vi "raster_scan_ground_shutter.vi"() -> ()   [LabVIEW 2013] (continued)
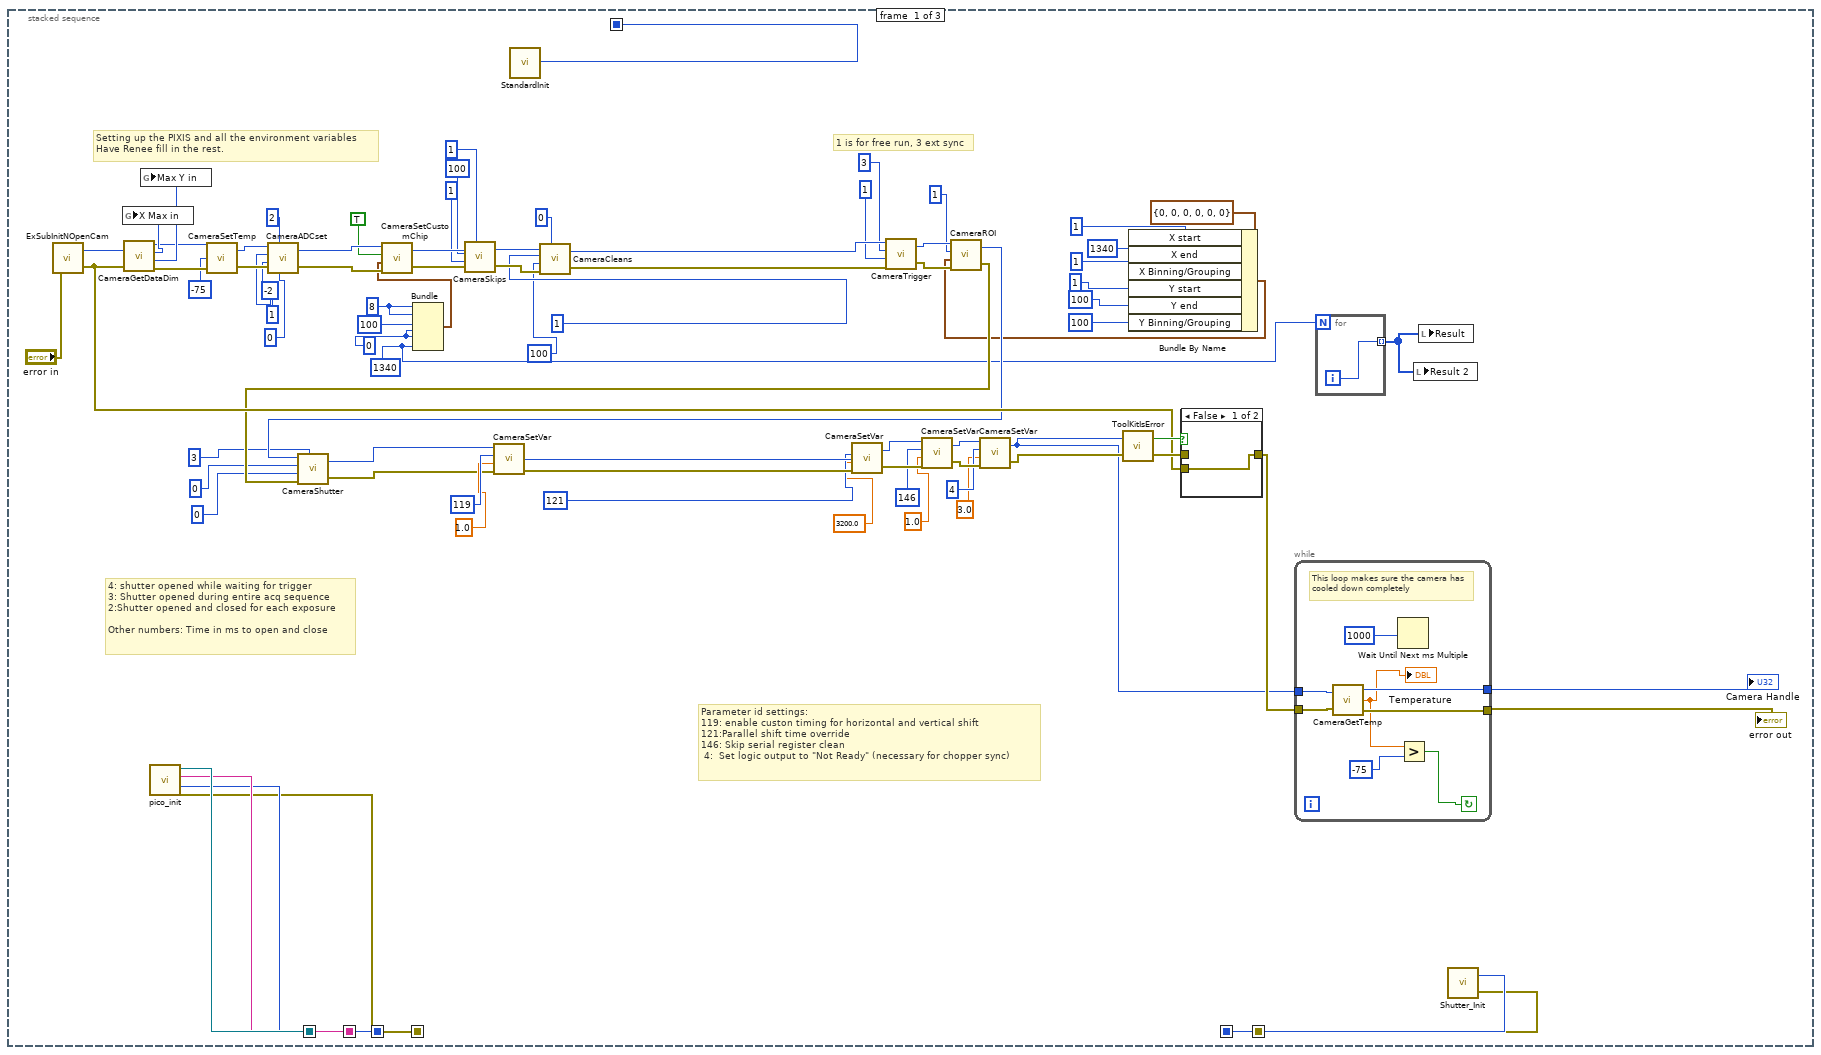
[diagram p2: hidden frame]
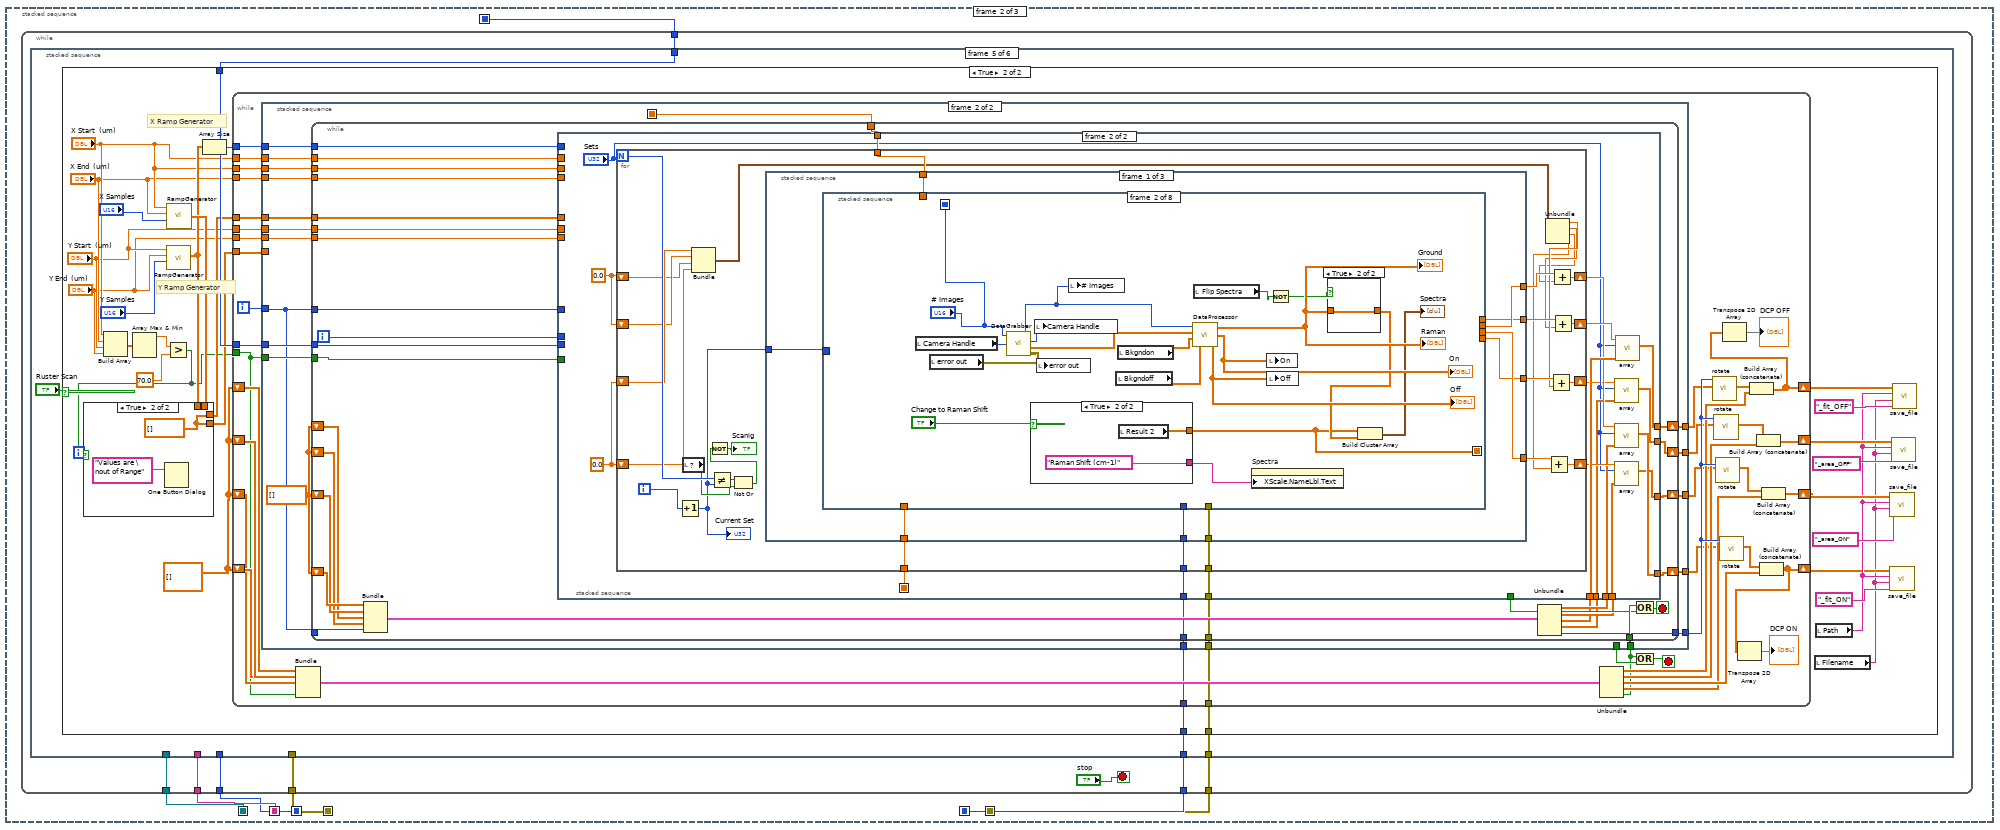
[diagram p4: hidden frame]
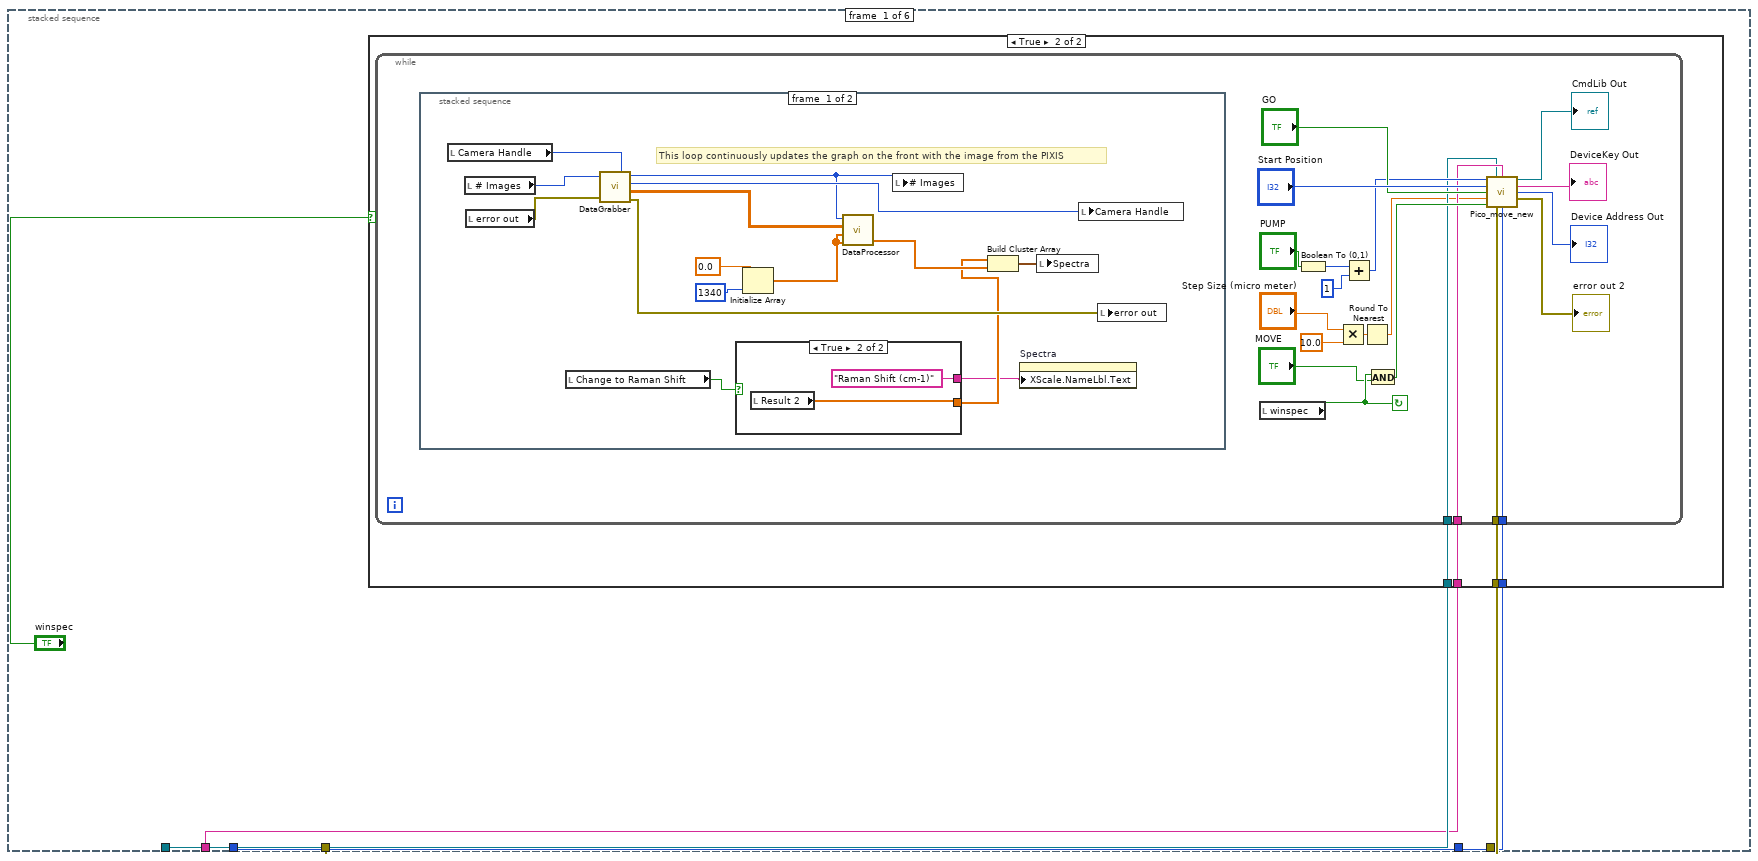
[diagram p5: hidden frame]
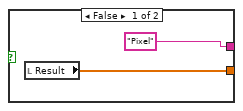
[diagram p7: hidden frame]
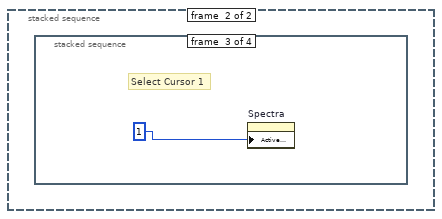
[diagram p8: hidden frame]
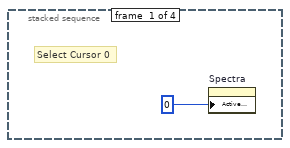
[diagram p9: hidden frame]
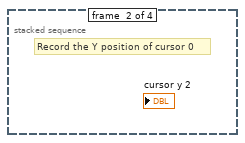
[diagram p10: hidden frame]
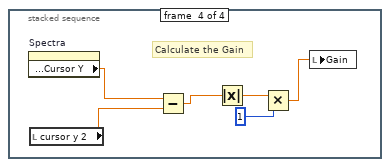
[diagram p11: hidden frame]
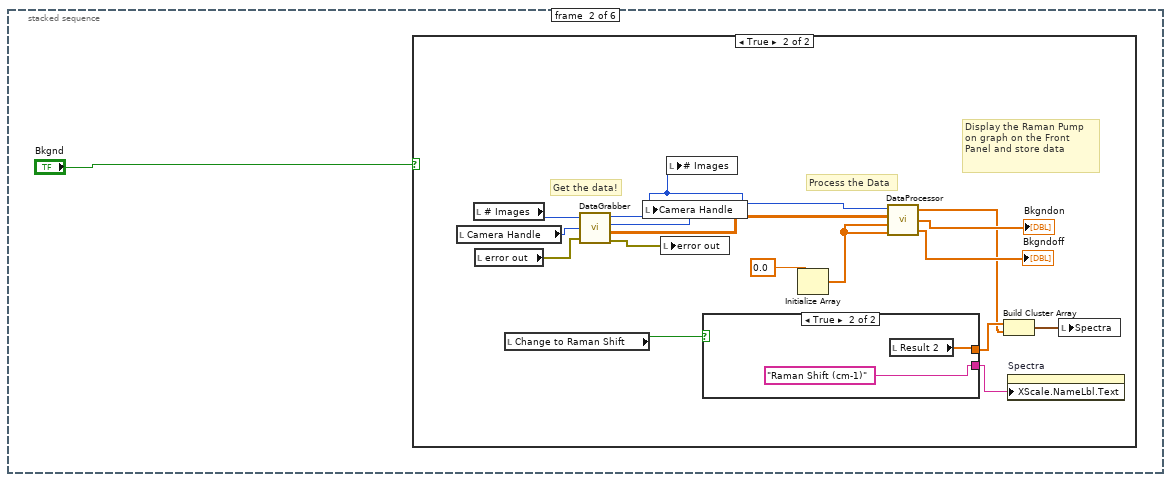
[diagram p12: hidden frame]
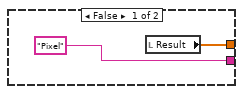
[diagram p14: hidden frame]
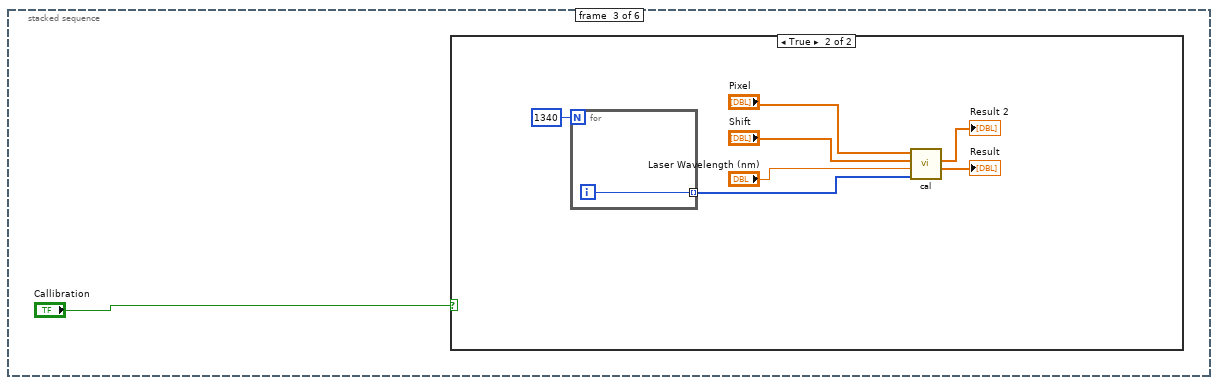
[diagram p15: hidden frame]
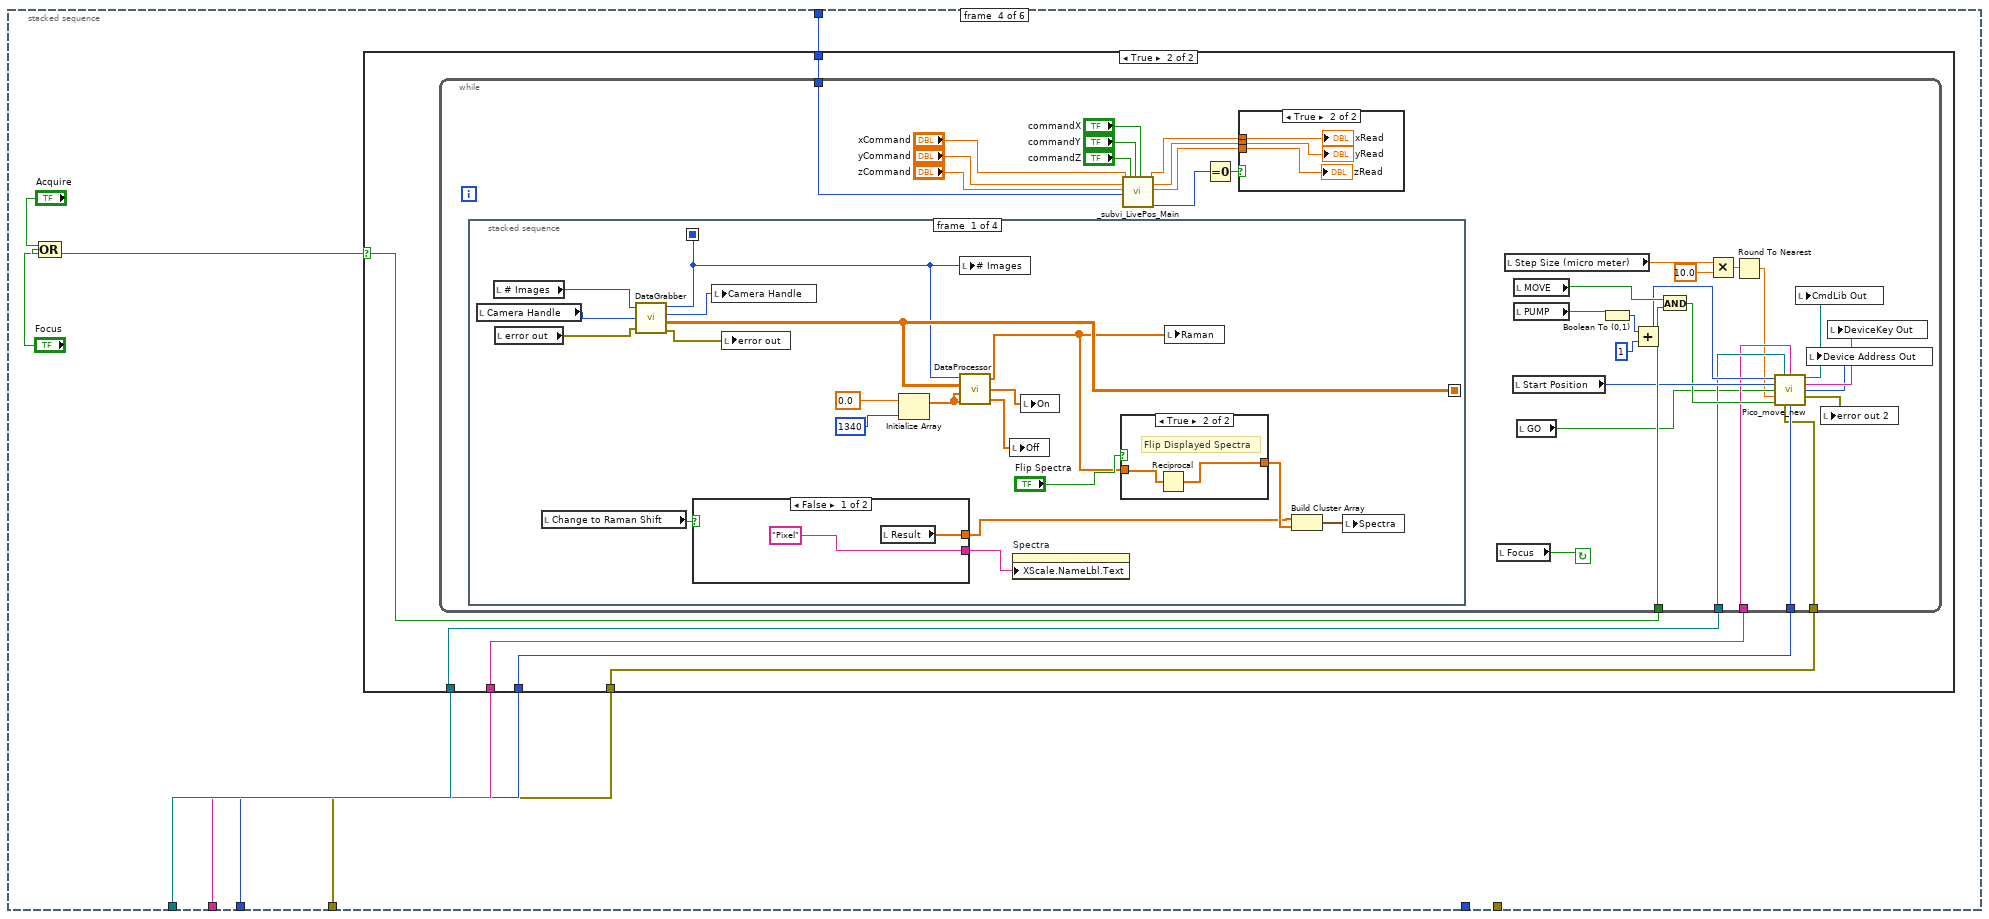
[diagram p17: hidden frame]
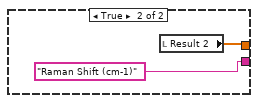
[diagram p20: hidden frame]
                  n154 = call "Pico_move_new.vi"("Motor"=w239, "CmdLib Out"=w236, "DeviceKey Out"=w235, "Start Position"=w238, "Boolean 2"=w232, "Relative Steps"=w224, "Boolean"=w237, "error out"=w233, "Device Address Out"=w234) -> ("CmdLib Out"=w231:refnum<k24>, "DeviceKey Out"=w230:string, "Device Address Out"=w229:i32, "error out 2"=w228:errorcluster)  [unwired: 3 in]
                  n155 = local write "CmdLib Out"(w231) -> ()
                  n156 = local write "Device Address Out"(w229) -> ()
                  n157 = local write "error out 2"(w228) -> ()
                  n158 = local write "DeviceKey Out"(w230) -> ()
                }
              }
            }
          }
          frame #4 {
            n159 = case shown="True" "Ruster Scan" {
              tunnel: w326 -> [_ w356]
              tunnel: w325 -> [_ w330]
              tunnel: w324 -> [_ w329]
              frame False {
              }
              frame True {
                w348 = dbl[][] []
                # "X Ramp Generator"
                # "Y Ramp Generator"
                n160 = Build Array("X Start  (um)", "X End  (um)", "Y Start  (um)", "Y End  (um)") -> (w347:dbl[])
                n161 = Array Max & Min(array=w347) -> (max value=w341:dbl)  [unwired: 3 out]
                n162 = call "RampGenerator.vi"("Number of Positions"="Y Samples", "End  (um)"="Y End  (um)", "Start  (um)"="Y Start  (um)") -> ("Array"=w350:dbl[])  [unwired: 1 in]
                n163 = Greater?(x=w341, y=70.0) -> (0:w331:bool)
                n164 = call "RampGenerator.vi"("Number of Positions"="X Samples", "End  (um)"="X End  (um)", "Start  (um)"="X Start  (um)") -> ("Array"=w351:dbl[])  [unwired: 1 in]
                n165 = case shown="True" w331 {
                  tunnel: [w358 w360] -> w352
                  tunnel: w350 -> [w358 _]
                  tunnel: [w357 w360] -> w353
                  tunnel: w351 -> [w357 _]
                  frame False {
                  }
                  frame True {
                    w360 = dbl[] [] ("Array")
                    n166 = One Button Dialog(message="Values are \nout of Range") -> ()  [unwired: 1 in, 1 out]
                  }
                }
                n167 = Array Size(array=w350) -> (size(s)=w349:i32)
                n168 = while {
                  tunnel: w352 -> [w400]
                  tunnel: w356 -> [w399]
                  tunnel: w353 -> [w398]
                  tunnel: "X Start  (um)" -> [w397]
                  shift-right: [w392] -> w332
                  shift-left: w348 -> [w375]
                  shift-right: [w394] -> w336
                  shift-left: w348 -> [w374]
                  tunnel: w331 -> [w365]
                  tunnel: w349 -> [w389]
                  tunnel: "X Start  (um)" -> [w388]
                  tunnel: "X End  (um)" -> [w387]
                  tunnel: "Y Start  (um)" -> [w386]
                  tunnel: "Y End  (um)" -> [w385]
                  shift-right: [w380] -> w337
                  shift-left: w348 -> [w376]
                  shift-right: [w378] -> w340
                  shift-left: w348 -> [w377]
                  tunnel: w330 -> [w362]
                  tunnel: w329 -> [w361]
                  i -> [w396]
                  stop <- w363 stop-if-true
                  n169 = Bundle(w377, w376, w375, w374, w365) -> (w373:T3)  [unwired: 1 in]
                  n170 = Unbundle(w373) -> (w372:dbl[][], w369:dbl[][], w371:dbl[][], w370:dbl[][], w364:bool)
                  n171 = stacked-sequence {
                    seq-local: [w402 _] -> [_ w428]
                    tunnel: w400 -> [w406 _]
                    tunnel: w396 -> [w404 w415]
                    tunnel: w399 -> [w405 w429]
                    tunnel: w398 -> [_ w431]
                    tunnel: w397 -> [_ w430]
                    tunnel: [w403 _] -> w391
                    tunnel: [_ w427] -> w368
                    tunnel: [_ w426] -> w367
                    tunnel: [_ w414] -> w384
                    tunnel: w365 -> [_ w425]
                    tunnel: w364 -> [_ w424]
                    tunnel: w389 -> [_ w423]
                    tunnel: w388 -> [_ w422]
                    tunnel: w387 -> [_ w421]
                    tunnel: w386 -> [_ w420]
                    tunnel: w385 -> [_ w419]
                    tunnel: [_ w417] -> w366
                    tunnel: [_ w416] -> w383
                    tunnel: w362 -> [_ w413]
                    tunnel: w361 -> [_ w412]
                    frame #0 {
                      w409 = 2  # Y AXIS
                      # "Step the Y axis"
                      n172 = Array Size(array=w406) -> (size(s)=w401:i32)
                      n173 = Index Array(array=w406, index=w404) -> (element=w407:dbl)
                      n174 = Increment(x=w404) -> (x+1=w408:i32)
                      n175 = Subtract(x=w401, y=w408) -> (x-y=w411:i32)
                      n176 = Equal To 0?(x=w411) -> (x = 0?=w403:bool)
                      n177 = call "WriteReadN.vi"("Handle"=w405, "Axis"=w409, "Delay (ms)"="Y Delay (ms)", "Move to (um)"=w407) -> ("Current Position (um)"=w402:dbl)
                      "Y Position (um)" <- w402
                    }
                    frame #1 {
                      w418 = dbl[] []
                      n178 = while {
                        tunnel: w431 -> [w463]
                        tunnel: w430 -> [w462]
                        tunnel: w429 -> [w460]
                        tunnel: w428 -> [w459]
                        tunnel: w415 -> [w446]
                        shift-right: [w458] -> w427
                        shift-left: w418 -> [w445]
                        shift-right: [w457] -> w426
                        shift-left: w418 -> [w444]
                        tunnel: w425 -> [w456]
                        tunnel: w424 -> [w454]
                        tunnel: w423 -> [w453]
                        tunnel: w422 -> [w452]
                        tunnel: w421 -> [w451]
                        tunnel: w420 -> [w450]
                        tunnel: w419 -> [w449]
                        shift-right: [w448] -> w417
                        shift-left: w418 -> [w443]
                        shift-right: [w447] -> w416
                        shift-left: w418 -> [w438]
                        tunnel: w415 -> [w435]
                        tunnel: [w434] -> w414
                        tunnel: w413 -> [w433]
                        tunnel: w412 -> [w432]
                        i -> [w461]
                        stop <- w455 stop-if-true
                        n179 = Bundle(w445, w444, w438, w443, w435) -> (w441:cluster{dbl[], dbl[], dbl[], dbl[], i32})  [unwired: 1 in]
                        n180 = Unbundle(w441) -> (w440:dbl[], w439:dbl[], w437:dbl[], w436:dbl[], w434:i32)
                        n181 = stacked-sequence {
                          seq-local: [w481 _] -> [_ w520]
                          tunnel: w463 -> [w486 _]
                          tunnel: w462 -> [_ _]
                          tunnel: w461 -> [w477 _]
                          tunnel: w460 -> [w494 _]
                          tunnel: [w493 _] -> w442
                          tunnel: w459 -> [w492 w521]
                          tunnel: w446 -> [w479 _]
                          tunnel: w440 -> [_ w512]
                          tunnel: [_ w511] -> w458
                          tunnel: [_ w505] -> w457
                          tunnel: w439 -> [_ w514]
                          tunnel: w456 -> [_ _]
                          tunnel: w453 -> [w480 _]
                          tunnel: w452 -> [w469 _]
                          tunnel: w451 -> [w468 _]
                          tunnel: w450 -> [w466 _]
                          tunnel: w449 -> [w467 _]
                          tunnel: w436 -> [_ w509]
                          tunnel: [_ w508] -> w448
                          tunnel: w437 -> [_ w517]
                          tunnel: [_ w515] -> w447
                          tunnel: w433 -> [_ w504]
                          tunnel: w432 -> [_ w503]
                          frame #0 {
                            w495 = 1  # X AXIS
                            # "Step the X axis"
                            n182 = Quotient & Remainder(x=w479, y=2) -> (x-y*floor(x/y)=w490:i32)  [unwired: 1 out]
                            n183 = Array Size(array=w486) -> (size(s)=w478:i32)
                            n184 = Equal?(x=w490, y=0) -> (x = y?=w483:bool)
                            n185 = Multiply(x=w478, y=w479) -> (x*y=w475:i32)
                            n186 = Increment(x=w477) -> (x+1=w476:i32)
                            n187 = Subtract(x=w478, y=1) -> (x-y=w484:i32)
                            n188 = Add(x=w475, y=w476) -> (x+y=w472:i32)
                            n189 = Multiply(x=w480, y=w478) -> (x*y=w471:i32)
                            n190 = Divide(x=w472, y=w471) -> (x/y=w474:dbl)
                            n191 = Subtract(x=w484, y=w477) -> (x-y=w487:i32)
                            n192 = case shown="False" w483 {
                              tunnel: w486 -> [w498 w502]
                              tunnel: w477 -> [_ w501]
                              tunnel: [w499 w500] -> w488
                              tunnel: w487 -> [w497 _]
                              frame False {
                                n193 = Index Array(array=w498, index=w497) -> (element=w499:dbl)
                              }
                              frame True {
                                n194 = Index Array(array=w502, index=w501) -> (element=w500:dbl)
                              }
                            }
                            n195 = Multiply(x=w474, y=100.0) -> (x*y=→"Progress (%)":dbl)
                            n196 = Equal To 0?(x=w487) -> (x = 0?=w493:bool)
                            n197 = Not Equal?(x=w471, y=w472) -> (x != y?=w465:bool)
                            "?" <- w465
                            n198 = call "WriteReadN.vi"("Handle"=w494, "Axis"=w495, "Delay (ms)"="X Deyal (ms)", "Move to (um)"=w488) -> ("Current Position (um)"=w481:dbl)
                            "X Position (um)" <- w481
                            n199 = Not(x=w465) -> (.not. x?=w470:bool)
                            n200 = call "?"("Reset"=w470, "Y Input"=w492, "X Input"=w481) -> ("XY Graph"=→"XY Graph":cluster{"X":dbl[], "Y":dbl[]}[])  [unwired: 7 in, 1 out]
                            n201 = property on="XY Graph" class="XYGraph (strict)"("XScale.Maximum"=w468) -> ()  [unwired: 2 in, 2 out]
                            n202 = property on="XY Graph" class="XYGraph (strict)"("YScale.Minimum"=w466) -> ()  [unwired: 2 in, 2 out]
                            n203 = property on="XY Graph" class="XYGraph (strict)"("YScale.Maximum"=w467) -> ()  [unwired: 2 in, 2 out]
                            n204 = property on="XY Graph" class="XYGraph (strict)"("XScale.Minimum"=w469) -> ()  [unwired: 2 in, 2 out]
                          }
                          frame #1 {
                            w518 = 0.0
                            w519 = 0.0
                            n205 = for {
                              N: "Sets" -> [w538]
                              tunnel: w520 -> [w548]
                              tunnel: w521 -> [w547]
                              shift-right: [w545] -> w510
                              shift-left: w519 -> [w533]
                              shift-right: [w544] -> w513
                              shift-left: w518 -> [w532]
                              shift-right: [w540] -> w516
                              shift-left: w519 -> [w534]
                              shift-right: [w539] -> w506
                              shift-left: w518 -> [w535]
                              tunnel: w504 -> [w525]
                              tunnel: w503 -> [w524]
                              i -> [w549]
                              n206 = Increment(x=w549) -> (x+1=w526:i32)
                              "Current Set" <- w526
                              n207 = local read item#71() -> (w536:bool)
                              n208 = Bundle(w535, w534, w533, w532) -> (w531:cluster{dbl, dbl, dbl, dbl})  [unwired: 1 in]
                              n209 = Not Equal?(x=w538, y=w526) -> (x != y?=w537:bool)
                              n210 = Not Or(1:w536, 2:w537) -> (0:w523:bool)
                              n211 = Not(x=w523) -> (.not. x?=→"Scanig":bool)
                              n212 = stacked-sequence {
                                tunnel: w526 -> [w550 _ _]
                                tunnel: w548 -> [w558 _ _]
                                tunnel: w547 -> [w557 _ _]
                                tunnel: [w556 _ _] -> w546
                                tunnel: [w555 _ _] -> w543
                                tunnel: [w554 _ _] -> w542
                                tunnel: [w553 _ _] -> w541
                                tunnel: w525 -> [w552 _ _]
                                tunnel: w524 -> [w551 _ _]
                                frame #0 {
                                n213 = stacked-sequence {
                                seq-local: [_ "# Images" _ _ _ _ _ _] -> [_ _ _ _ _ w640 _ _]
                                seq-local: [_ w566 _ _ _ _ _ _] -> [_ _ w592 _ _ _ w658 _]
                                tunnel: w558 -> [_ _ _ w614 _ _ _ w678]
                                tunnel: w557 -> [_ _ _ w613 _ _ _ w677]
                                tunnel: [_ _ w594 _ _ _ _ _] -> w556
                                tunnel: [_ _ w593 _ _ _ _ _] -> w555
                                tunnel: w550 -> [_ _ _ w615 _ _ _ w679]
                                tunnel: [_ _ _ _ _ _ w657 _] -> w554
                                tunnel: [_ _ _ _ _ _ w656 _] -> w553
                                tunnel: w552 -> [w560 _ _ _ w624 _ _ _]
                                tunnel: w551 -> [w559 _ _ _ w623 _ _ _]
                                frame #0 {
                                n214 = flat-sequence {
                                tunnel: w560 -> [w564]
                                tunnel: w559 -> [w563]
                                frame #0 {
                                n215 = call "shutter_new.vi"("error in"=w563, "ShutterID"=310, "Shutter Position"=TRUE, "ObjectPtr"=w564) -> ()  [unwired: 1 out]
                                }
                                frame #1 {
                                n216 = Wait (ms)(milliseconds to wait=u32 200) -> ()  [unwired: 1 out]
                                }
                                }
                                }
                                frame #1 {
                                n217 = local read "Camera Handle"() -> (w584:u32)
                                n218 = local read "error out"() -> (w583:errorcluster)
                                n219 = call "DataGrabber.vi"("# Images In"="# Images", "Camera Handle"=w584, "error in (no error)"=w583) -> ("# Images Out"=w577:u16, "Camera Handle"=w581:u32, "Data"=w580:dbl[][], "error out"=w582:errorcluster)
                                n220 = case shown="True" "Change to Raman Shift" {
                                tunnel: [w586 w588] -> w566
                                tunnel: ["Pixel" ("X Scale.Name Label.Text") "Raman Shift (cm-1)" ("X Scale.Name Label.Text")] -> w569
                                frame False {
                                n221 = local read "Result"() -> (w586:dbl[])
                                }
                                frame True {
                                n222 = local read "Result 2"() -> (w588:dbl[])
                                }
                                }
                                n223 = local write "Camera Handle"(w581) -> ()
                                n224 = local write "error out"(w582) -> ()
                                n225 = local write "# Images"(w577) -> ()
                                n226 = local read "Bkgndoff"() -> (w578:dbl[])
                                n227 = local read "Bkgndon"() -> (w579:dbl[])
                                n228 = call "DataProcessor.vi"("PumpOffBkgd"=w578, "PumpOnBkgd"=w579, "Data"=w580, "# of Images"=w577) -> ("PumpOff"=w575:dbl[], "PumpOn"=w574:dbl[], "Raman"=w573:dbl[])
                                "Ground" <- w573
                                "On" <- w574
                                "Off" <- w575
                                "Raman" <- w573
                                n229 = local read "Flip Spectra"() -> (w568:bool)
                                n230 = property on="Spectra" class="XYGraph (strict)"("XScale.NameLbl.Text"=w569) -> ()  [unwired: 2 in, 2 out]
                                n231 = local write "On"(w574) -> ()
                                n232 = local write "Off"(w575) -> ()
                                n233 = Not(x=w568) -> (.not. x?=w567:bool)
                                n234 = case shown="True" w567 {
                                tunnel: w573 -> [w589 w591]
                                tunnel: [w590 w591] -> w572
                                frame False {
                                n235 = Reciprocal(x=w589) -> (1/x=w590:dbl[])
                                }
                                frame True {
                                }
                                }
                                n236 = Build Cluster Array(w566, w572) -> (→"Spectra":cluster{dbl, dbl}[])
                                }
                                frame #2 {
                                # "Peak fitting and intergation"
                                n237 = local read "Raman"() -> (w596:dbl[])
                                n238 = property on="Spectra" class="XYGraph (strict)"("Active Cursor"=u32 1) -> ("Cursor.Cursor X"=w598:dbl)  [unwired: 2 in, 2 out]
                                n239 = property on="Spectra" class="XYGraph (strict)"("Active Cursor"=u32 0) -> ("Cursor.Cursor X"=w599:dbl)  [unwired: 2 in, 2 out]
                                n240 = call "fit_new.vi"("Cursor1 2"=w598, "Cursor1"=w599, "array 2"=w592, "array"=w596, "Fano Fit ?"="Fano Fit ?", "Fano initial Parameters"="Fano initial Parameters") -> ("Intergrate"=w593:dbl, "Fit"=w594:dbl)  [unwired: 4 in]
                                "FIT" <- w594
                                "AREA" <- w593
                                }
                                frame #3 {
                                # "Here we save spectrum for each special point"
                                n241 = Format Into String(w615) -> (resulting string=w607:string)  [unwired: 3 in, 1 out]
                                n242 = call "number_to_sring.vi"("Numeric"=w614) -> ("result string"=w605:string)  [unwired: 10 in]
                                n243 = call "number_to_sring.vi"("Numeric"=w613) -> ("result string"=w603:string)  [unwired: 10 in]
                                n244 = Concatenate Strings("Path", "\\", "Filename", "_", w607, "_X_" ("string"), w605, "_Y_" ("string"), w603, "_ON" ("string")) -> (w612:string)
                                "File_name" <- w612
                                n245 = local read "Ground"() -> (w618:dbl[])
                                n246 = local read "On"() -> (w622:dbl[])
                                n247 = local read "Off"() -> (w621:dbl[])
                                n248 = String To Path(string=w612) -> (path=w619:path)
                                n249 = Build Array(w618, w622, w621) -> (w620:dbl[][])
                                n250 = call-poly <vilib>:"Write To Spreadsheet File.vi"("transpose? (no:F)"=TRUE, "format (%.3f)"="%.7f", "2D data"=w620, "file path (dialog if empty)"=w619) -> ()  [unwired: 4 in, 1 out]
                                }
                                frame #4 {
                                n251 = flat-sequence {
                                tunnel: w624 -> [w628]
                                tunnel: w623 -> [w627]
                                frame #0 {
                                n252 = call "shutter_new.vi"("error in"=w627, "ShutterID"=310, "Shutter Position"=FALSE, "ObjectPtr"=w628) -> ()  [unwired: 1 out]
                                }
                                frame #1 {
                                n253 = Wait (ms)(milliseconds to wait=u32 200) -> ()  [unwired: 1 out]
                                }
                                }
                                }
                                frame #5 {
                                n254 = local read "Camera Handle"() -> (w648:u32)
                                n255 = local read "error out"() -> (w647:errorcluster)
                                n256 = local read "Change to Raman Shift"() -> (w635:bool)
                                n257 = call "DataGrabber.vi"("# Images In"=w640, "Camera Handle"=w648, "error in (no error)"=w647) -> ("# Images Out"=w641:u16, "Camera Handle"=w645:u32, "Data"=w644:dbl[][], "error out"=w646:errorcluster)
                                n258 = local write "Camera Handle"(w645) -> ()
                                n259 = local write "error out"(w646) -> ()
                                n260 = local write "# Images"(w641) -> ()
                                n261 = local read "Bkgndoff"() -> (w642:dbl[])
                                n262 = local read "Bkgndon"() -> (w643:dbl[])
                                n263 = case shown="False" w635 {
                                tunnel: [w650 w652] -> w634
                                tunnel: ["Pixel" ("X Scale.Name Label.Text") "Raman Shift (cm-1)" ("X Scale.Name Label.Text")] -> w636
                                frame False {
                                n264 = local read "Result"() -> (w650:dbl[])
                                }
                                frame True {
                                n265 = local read "Result 2"() -> (w652:dbl[])
                                }
                                }
                                n266 = call "DataProcessor.vi"("PumpOffBkgd"=w642, "PumpOnBkgd"=w643, "Data"=w644, "# of Images"=w641) -> ("PumpOff"=w639:dbl[], "PumpOn"=w638:dbl[], "Raman"=w637:dbl[])
                                n267 = local read "Flip Spectra"() -> (w631:bool)
                                n268 = Not(x=w631) -> (.not. x?=w630:bool)
                                n269 = local write "On"(w638) -> ()
                                n270 = local write "Off"(w639) -> ()
                                n271 = case shown="True" w630 {
                                tunnel: w637 -> [w654 w655]
                                tunnel: [w653 w655] -> w633
                                frame False {
                                n272 = Reciprocal(x=w654) -> (1/x=w653:dbl[])
                                }
                                frame True {
                                }
                                }
                                n273 = property on="Spectra" class="XYGraph (strict)"("XScale.NameLbl.Text"=w636) -> ()  [unwired: 2 in, 2 out]
                                n274 = local write "Ground"(w637) -> ()
                                n275 = local write "Raman"(w637) -> ()
                                n276 = Build Cluster Array(w634, w633) -> (w632:cluster{dbl, dbl}[])
                                n277 = local write "Off"(w639) -> ()
                                n278 = local write "Spectra"(w632) -> ()
                                n279 = local write "On"(w638) -> ()
                                }
                                frame #6 {
                                # "Peak fitting and intergation"
                                n280 = local read "Fano initial Parameters"() -> (w660:T1)
                                n281 = local read "Fano Fit ?"() -> (w661:bool)
                                n282 = local read "Raman"() -> (w659:dbl[])
                                n283 = property on="Spectra" class="XYGraph (strict)"("Active Cursor"=u32 0) -> ("Cursor.Cursor X"=w663:dbl)  [unwired: 2 in, 2 out]
                                n284 = property on="Spectra" class="XYGraph (strict)"("Active Cursor"=u32 1) -> ("Cursor.Cursor X"=w662:dbl)  [unwired: 2 in, 2 out]
                                n285 = call "fit_new.vi"("Cursor1 2"=w662, "Cursor1"=w663, "array 2"=w658, "array"=w659, "Fano Fit ?"=w661, "Fano initial Parameters"=w660) -> ("Intergrate"=w656:dbl, "Fit"=w657:dbl)  [unwired: 4 in]
                                n286 = local write "AREA"(w656) -> ()
                                n287 = local write "FIT"(w657) -> ()
                                }
                                frame #7 {
                                # "Here we save spectrum for each special point"
                                n288 = local read "Filename"() -> (w673:string)
                                n289 = local read "Path"() -> (w675:string)
                                n290 = Format Into String(w679) -> (resulting string=w671:string)  [unwired: 3 in, 1 out]
                                n291 = call "number_to_sring.vi"("Numeric"=w678) -> ("result string"=w669:string)  [unwired: 10 in]
                                n292 = call "number_to_sring.vi"("Numeric"=w677) -> ("result string"=w667:string)  [unwired: 10 in]
                                n293 = Concatenate Strings(w675, "\\", w673, "_", w671, "_X_" ("string"), w669, "_Y_" ("string"), w667, "_OFF" ("string")) -> (w676:string)
                                n294 = local read "Ground"() -> (w682:dbl[])
                                n295 = local read "Off"() -> (w686:dbl[])
                                n296 = local read "Off"() -> (w685:dbl[])
                                n297 = String To Path(string=w676) -> (path=w683:path)
                                n298 = local write "File_name"(w676) -> ()
                                n299 = Build Array(w682, w686, w685) -> (w684:dbl[][])
                                n300 = call-poly <vilib>:"Write To Spreadsheet File.vi"("transpose? (no:F)"=TRUE, "format (%.3f)"="%.7f", "2D data"=w684, "file path (dialog if empty)"=w683) -> ()  [unwired: 4 in, 1 out]
                                }
                                }
                                }
                                frame #1 {
                                n301 = stacked-sequence {
                                frame #0 {
                                n302 = property on="Spectra" class="XYGraph (strict)"("Active Cursor"=0) -> ()  [unwired: 2 in, 2 out]
                                }
                                frame #1 {
                                n303 = property on="Spectra" class="XYGraph (strict)"() -> ("Cursor.Cursor Position:Cursor Y"=w688:dbl)  [unwired: 2 in, 2 out]
                                n304 = local write "cursor y"(w688) -> ()
                                }
                                frame #2 {
                                n305 = property on="Spectra" class="XYGraph (strict)"("Active Cursor"=1) -> ()  [unwired: 2 in, 2 out]
                                }
                                frame #3 {
                                n306 = property on="Spectra" class="XYGraph (strict)"() -> ("Cursor.Cursor Position:Cursor Y"=w690:dbl)  [unwired: 2 in, 2 out]
                                n307 = local read "cursor y"() -> (w691:dbl)
                                n308 = Subtract(x=w690, y=w691) -> (x-y=w693:dbl)
                                n309 = Absolute Value(x=w693) -> (abs(x)=w695:dbl)
                                n310 = Multiply(x=w695, y=100) -> (x*y=w692:dbl)
                                n311 = local write "Gain"(w692) -> ()
                                }
                                }
                                }
                                frame #2 {
                                n312 = while {
                                stop <- "Pause" continue-if-true
                                }
                                }
                              }
                              n313 = Unbundle(w531) -> (w530:dbl, w529:dbl, w528:dbl, w527:dbl)
                              n314 = Add(x=w543, y=w527) -> (x+y=w544:dbl)
                              n315 = Add(x=w541, y=w530) -> (x+y=w539:dbl)
                              n316 = Add(x=w546, y=w528) -> (x+y=w545:dbl)
                              n317 = Add(x=w542, y=w529) -> (x+y=w540:dbl)
                            }
                            n318 = call "array.vi"("x"=w506, "y"="Sets", "array"=w509) -> ("appended array"=w508:dbl[])  [unwired: 6 in]
                            n319 = call "array.vi"("x"=w510, "y"="Sets", "array"=w512) -> ("appended array"=w511:dbl[])  [unwired: 6 in]
                            n320 = call "array.vi"("x"=w513, "y"="Sets", "array"=w514) -> ("appended array"=w505:dbl[])  [unwired: 6 in]
                            n321 = call "array.vi"("x"=w516, "y"="Sets", "array"=w517) -> ("appended array"=w515:dbl[])  [unwired: 6 in]
                          }
                        }
                        n322 = Or(x=w454, y=w442) -> (x .or. y?=w455:bool)
                      }
                    }
                  }
                  n323 = Or(x=w364, y=w391) -> (x .or. y?=w363:bool)
                  n324 = call "rotate.vi"("Array in"=w383, "i"=w384) -> ("Array out"=w381:dbl[])  [unwired: 9 in]
                  n325 = call "rotate.vi"("Array in"=w366, "i"=w384) -> ("Array out"=w382:dbl[])  [unwired: 9 in]
                  n326 = call "rotate.vi"("Array in"=w367, "i"=w384) -> ("Array out"=w395:dbl[])  [unwired: 9 in]
                  n327 = call "rotate.vi"("Array in"=w368, "i"=w384) -> ("Array out"=w393:dbl[])  [unwired: 9 in]
                  n328 = Build Array (concatenate)(w381, w372) -> (w378:dbl[][])
                  n329 = Transpose 2D Array(2D array=w378) -> (transposed array=→"DCP OFF":dbl[][])
                  n330 = Build Array (concatenate)(w382, w369) -> (w380:dbl[][])
                  n331 = Build Array (concatenate)(w393, w371) -> (w392:dbl[][])
                  n332 = Transpose 2D Array(2D array=w392) -> (transposed array=→"DCP ON":dbl[][])
                  n333 = Build Array (concatenate)(w395, w370) -> (w394:dbl[][])
                }
                n334 = local read "Filename"() -> (w328:string)
                n335 = local read "Path"() -> (w333:string)
                n336 = call "save_file.vi"("string 3"="_area_ON" ("string"), "string 2"=w328, "string"=w333, "2D data"=w336) -> ()  [unwired: 8 in]
                n337 = call "save_file.vi"("string 3"="_fit_ON" ("string"), "string 2"=w328, "string"=w333, "2D data"=w332) -> ()  [unwired: 8 in]
                n338 = call "save_file.vi"("string 3"="_area_OFF" ("string"), "string 2"=w328, "string"=w333, "2D data"=w337) -> ()  [unwired: 8 in]
                n339 = call "save_file.vi"("string 3"="_fit_OFF" ("string"), "string 2"=w328, "string"=w333, "2D data"=w340) -> ()  [unwired: 8 in]
              }
            }
          }
          frame #5 {
            n340 = case shown="True" "Save" {
              frame False {
              }
              frame True {
                n341 = local read "Raman"() -> (w720:dbl[])
                n342 = local read "Off"() -> (w718:dbl[])
                n343 = local read "On"() -> (w719:dbl[])
                n344 = local read "Path"() -> (w717:string)
                n345 = Build Array(w720, w719, w718) -> (w711:dbl[][])
                n346 = local read "Filename"() -> (w715:string)
                n347 = Concatenate Strings(w717, "\\", w715) -> (w714:string)
                n348 = String To Path(string=w714) -> (path=w710:path)
                n349 = call-poly <vilib>:"Write To Spreadsheet File.vi"("transpose? (no:F)"=TRUE, "format (%.3f)"="%.7f", "2D data"=w711, "file path (dialog if empty)"=w710) -> ()  [unwired: 4 in, 1 out]
              }
            }
            n350 = case shown="True" "subtract" {
              frame False {
              }
              frame True {
                n351 = local read "Change to Raman Shift"() -> (w728:bool)
                n352 = local read "Subtrarray"() -> (w732:dbl[])
                n353 = local read "Raman"() -> (w731:dbl[])
                n354 = Multiply(x="Scale factor", y=w732) -> (x*y=w730:dbl[])
                n355 = Subtract(x=w731, y=w730) -> (x-y=w726:dbl[])
                n356 = case shown="True" w728 {
                  tunnel: [w735 w737] -> w727
                  tunnel: ["Pixel" ("X Scale.Name Label.Text") "Raman Shift (cm-1)" ("X Scale.Name Label.Text")] -> w729
                  frame False {
                    n357 = local read "Result"() -> (w735:dbl[])
                  }
                  frame True {
                    n358 = local read "Result 2"() -> (w737:dbl[])
                  }
                }
                n359 = property on="Spectra" class="XYGraph (strict)"("XScale.NameLbl.Text"=w729) -> ()  [unwired: 2 in, 2 out]
                n360 = Build Cluster Array(w727, w726) -> (w725:cluster{dbl, dbl}[])
                n361 = local write "Spectra"(w725) -> ()
              }
            }
            n362 = case shown="True" "ChooseBkgdFile" {
              frame False {
              }
              frame True {
                n363 = call-poly <vilib>:"Read From Spreadsheet File.vi"("transpose (no:F)"=TRUE) -> ("first row"=w739:dbl[], "new file path (Not A Path if cancelled)"=→"Background File":path)  [unwired: 6 in, 3 out]
                n364 = Array Subset(array=w739, index=0, length=1340) -> (→"Subtrarray":dbl[])
              }
            }
            n365 = case shown="True" "SetPath" {
              frame False {
              }
              frame True {
                (unwired) 5
                n366 = File Dialog(11:path "C:/DATA") -> (0:w721:errorcluster, 3:w724:path)  [unwired: 6 in, 2 out]
                n367 = Unbundle(w721) -> ()  [unwired: 3 out]
                n368 = Path To String(path=w724) -> (string=w722:string)
                n369 = local write "Path"(w722) -> ()
              }
            }
            n370 = case shown="True" "Boolean" {
              frame False {
              }
              frame True {
                n371 = local read "Path"() -> (w706:string)
                n372 = local read "Filename"() -> (w708:string)
                n373 = Concatenate Strings(w706, "\\", w708) -> (w709:string)
                n374 = String To Path(string=w709) -> (path=w705:path)
                n375 = local read "Off"() -> (w702:dbl[])
                n376 = call-poly <vilib>:"Write To Spreadsheet File.vi"("transpose? (no:F)"=TRUE, "format (%.3f)"="%.7f", "1D data"=w702, "file path (dialog if empty)"=w705) -> ()  [unwired: 4 in, 1 out]
              }
            }
          }
        }
      }
    }
    frame #2 {
      n377 = local read "DeviceKey Out"() -> (w746:string)
      n378 = local read "error out 2"() -> (w745:errorcluster)
      n379 = local read "CmdLib Out"() -> (w747:refnum<k24>)
      n380 = stacked-sequence {
        frame #0 {
          n381 = local read "Camera Handle"() -> (w748:u32)
          n382 = local read "error out"() -> (w749:errorcluster)
          n383 = call <userlib>:"CameraClose.vi"("error in"=w749, "Camera Handle"=w748) -> ("error out"=w751:errorcluster)
          n384 = call <userlib>:"UninitToolkit.vi"("error in"=w751) -> ("error out"=w750:errorcluster)
          n385 = local write "error out"(w750) -> ()
        }
      }
      n386 = call <instrlib>:"DeviceClose.vi"("error in (no error)"=w745, "DeviceKey In"=w746, "CmdLib In"=w747) -> ()  [unwired: 2 in, 3 out]
      n387 = dll-call lib="C:/Program Files/Mad City Labs/NanoDrive/Labview Examples/MADLib.dll" fn="MCL_ReleaseHandle"("handle"=w744) -> ()  [unwired: 5 in, 2 out]
    }
  }
